vi "Sorted Calibration Points.vi"(8 "error in (no error)":errorcluster, 10 "Linearity Descriptors":T1(array[cluster])=[{"Direction"="Acsending", "Cycle Number"=0, "SensorID"=18}, {"Direction"="Descending", "Cycle Number"=0, "SensorID"=18}, {"Direction"="Acsending", "Cycle Number"=1, "SensorID"=18}, {"Direction"="Descending", "Cycle Number"=1, "SensorID"=18}, {"Direction"="Acsending", "Cycle Number"=0, "SensorID"=22}, {"Direction"="Descending", "Cycle Number"=0, "SensorID"=22}, {"Direction"="Acsending", "Cycle Number"=1, "SensorID"=22}, {"Direction"="Descending", "Cycle Number"=1, "SensorID"=22}], 11 "Calibration Points":T2[](array[typedef])) -> (0 "error out":errorcluster, 3 "Sorted Calibration Points":T2[][](array[typedef]))   [LabVIEW 2026, in "Analysis.lvlib"]
uses:
  Analysis.lvlib
  controls/Messaging Payloads/Calibration Point Table Insert.ctl
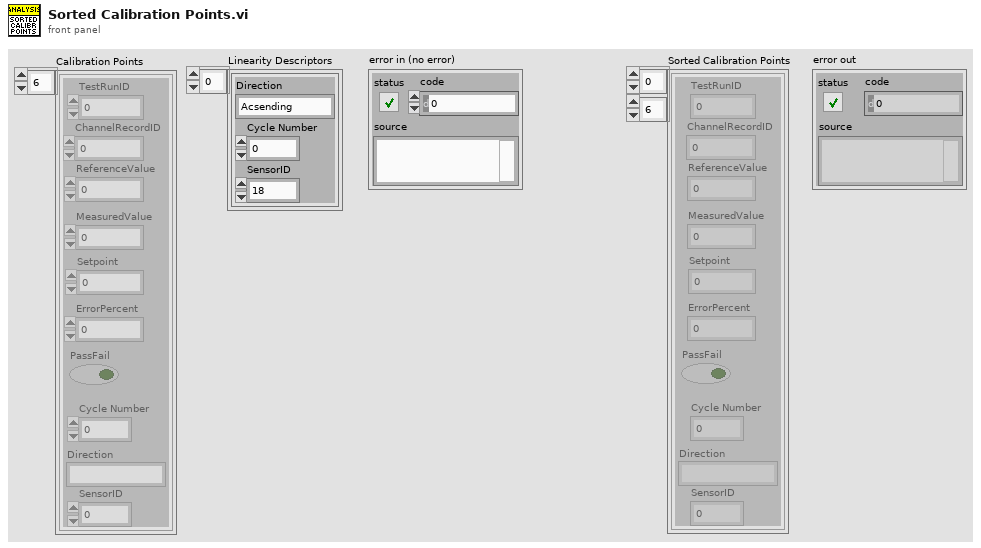
[diagram p1: front panel]
types:
  T1 = cluster{"Direction":string, "Cycle Number":i32, "SensorID":i32}[]
  T2 = typedef "Calibration Point Table Insert.ctl" = cluster{"TestRunID":i32, "ChannelRecordID":i32, "Setpoint":dbl, "MeasuredValue":dbl, "ErrorPercent":dbl, "PassFail":bool, "ReferenceValue":dbl, "Cycle Number":i32, "Direction":string, "SensorID":i32}
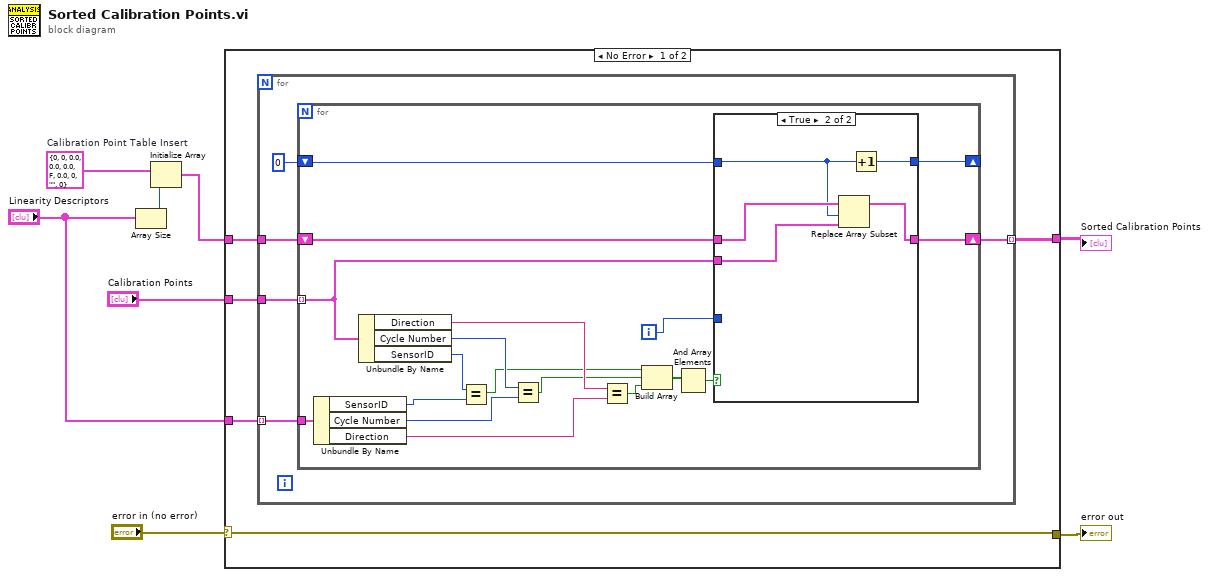
[diagram p0: block diagram]
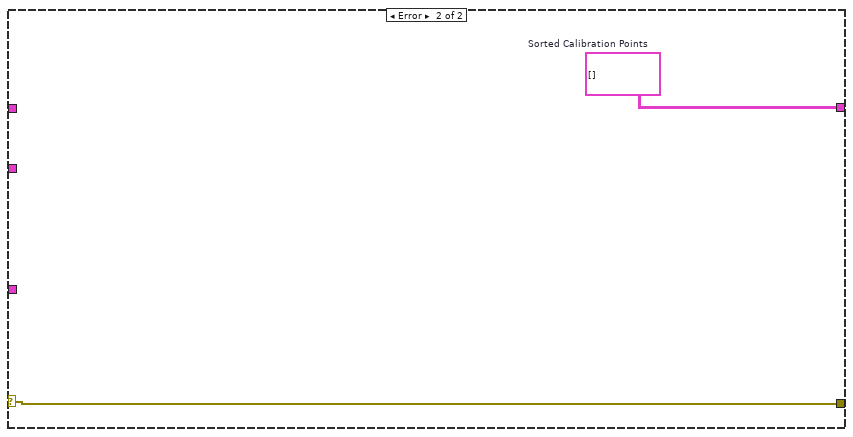
[diagram p3: hidden frame]
diagram:
  w4 = T2 {"TestRunID"=0, "ChannelRecordID"=0, "Setpoint"=0.0, "MeasuredValue"=0.0, "ErrorPercent"=0.0, "PassFail"=FALSE, "ReferenceValue"=0.0, "Cycle Number"=0, "Direction"="", "SensorID"=0}  # Calibration Point Table Insert
  n1 = Array Size(array="Linearity Descriptors") -> (size(s)=w2:i32)
  n2 = Initialize Array(w4, w2) -> (w1:T2[])
  n3 = case shown="No Error" "error in (no error)" {
    selector: "error in (no error)" -> [w13 w45]
    tunnel: "Calibration Points" -> [w9 _]
    tunnel: [w13 w45] -> w8
    tunnel: w1 -> [w11 _]
    tunnel: [w12 w44] -> w5
    tunnel: "Linearity Descriptors" -> [w10 _]
    frame No Error {
      n4 = for {
        tunnel: [w18] -> w12 mode=indexing
        tunnel: w11 -> [w17]
        tunnel: w10 -> [w16] mode=indexing
        tunnel: w9 -> [w14]
        n5 = for {
          tunnel: w14 -> [w27] mode=indexing
          shift-right: [w26] -> w18
          shift-left: w17 -> [w28]
          tunnel: w16 -> [w25]
          shift-right: [w21] -> _
          shift-left: 0 -> [w20]
          i -> [w19]
          n6 = Unbundle By Name(w25) -> ("SensorID"=w24:i32, "Cycle Number"=w23:i32, "Direction"=w22:string)
          n7 = Unbundle By Name(w27) -> ("Direction"=w34:string, "Cycle Number"=w35:i32, "SensorID"=w36:i32)
          n8 = Equal?(x=w36, y=w24) -> (x = y?=w31:bool)
          n9 = Equal?(x=w35, y=w23) -> (x = y?=w32:bool)
          n10 = Equal?(x=w34, y=w22) -> (x = y?=w33:bool)
          n11 = Build Array(w31, w32, w33) -> (w30:bool[])
          n12 = And Array Elements(Boolean array=w30) -> (logical AND=w29:bool)
          n13 = case shown="True" w29 {
            tunnel: w27 -> [_ w42]
            tunnel: [w38 w41] -> w26
            tunnel: w28 -> [w38 w43]
            tunnel: [w37 w39] -> w21
            tunnel: w20 -> [w37 w40]
            tunnel: w19 -> [_ _]
            frame False {
            }
            frame True {
              n14 = Replace Array Subset(array=w43, new element=w42, index=w40) -> (w41:T2[])
              n15 = Increment(x=w40) -> (x+1=w39:i32)
            }
          }
        }
      }
    }
    frame Error {
      w44 = T2[][] []  # Sorted Calibration Points
    }
  }
  "error out" <- w8
  "Sorted Calibration Points" <- w5
